vi "Airpuff.vi"() -> ()   [LabVIEW 2013]
uses:
  <vilib>/DAQmx/create/channels.llb/DAQmx Create Channel (DO-Digital Output).vi
panel:
  in  "Trigger Duration (ms)":u32=500
  in  "Quit Program":bool
  in  "lines":tag
  in  "Airpuff":bool
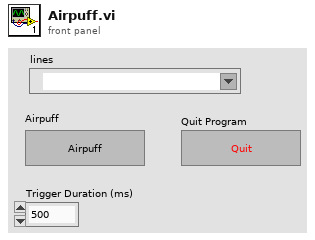
[diagram p1: front panel]
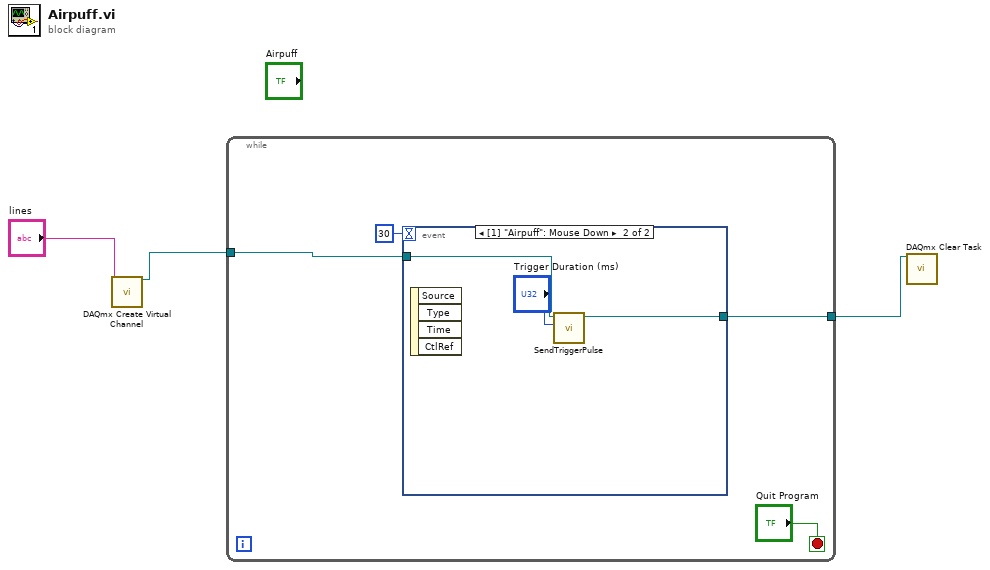
[diagram p0: block diagram]
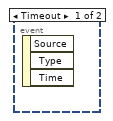
[diagram p2: hidden frame]
diagram:
  n1 = call-poly <vilib>:"DAQmx Create Virtual Channel.vi"("lines"="lines") -> ("task out"=w2:refnum<k21>)  [unwired: 13 in, 1 out]
  n2 = while {
    tunnel: w2 -> [w6]
    tunnel: [w5] -> w1
    stop <- "Quit Program" stop-if-true
    n3 = event shown="[1] \"Airpuff\": Mouse Down" {
      selector: _ -> [_ _]
      dyn-events: _ -> [_ _]
      timeout: 30 -> [_ _]
      tunnel: w6 -> [_ w9]
      tunnel: [_ w8] -> w5
      event Timeout {
        n4 = event-data() -> ()  [unwired: 1 in, 3 out]
      }
      event "Airpuff": Mouse Down {
        n5 = event-data() -> ()  [unwired: 1 in, 4 out]
        n6 = call "SendTriggerPulse.vi"("Trigger Duration (ms)"="Trigger Duration (ms)", "Refnum in"=w9) -> ("Refnum out"=w8:refnum<k21>)  [unwired: 9 in]
      }
    }
  }
  n7 = call <vilib>:"DAQmx Clear Task.vi"("task in"=w1) -> ()  [unwired: 14 in, 1 out]
